vi "UpdateVariablesTC.vi"(8 "error in (no error)":errorcluster, 9 "SignificantDigits (8)":u32=8, 10 "Format (SI notation)":T1(ring)=enum."SI notation", 11 "VMUI in":refnum<class "VMUI.lvclass">) -> (0 "error out":errorcluster, 3 "VMUI out":refnum<class "VMUI.lvclass">)   [LabVIEW 2013, in "VMUI.lvclass"]
uses:
  VMUI.lvclass
  VariableManager/VariableManager.lvclass
  API/VariableManagerAPI.lvlib
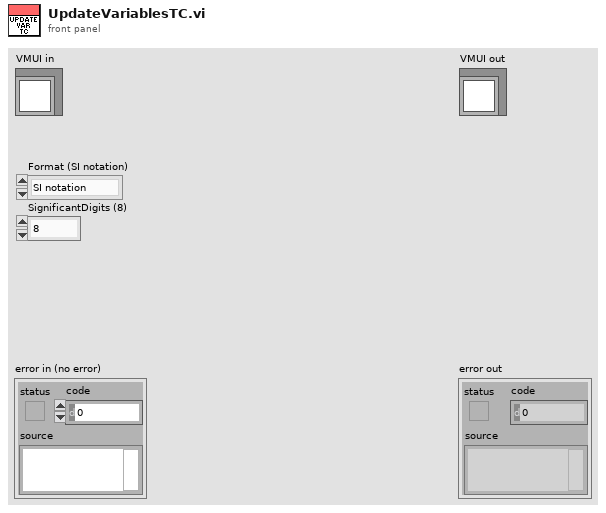
[diagram p1: front panel]
types:
  T1 = enum16{"Floating point", "Scientific SI", "Automatic SI", "SI notation"}
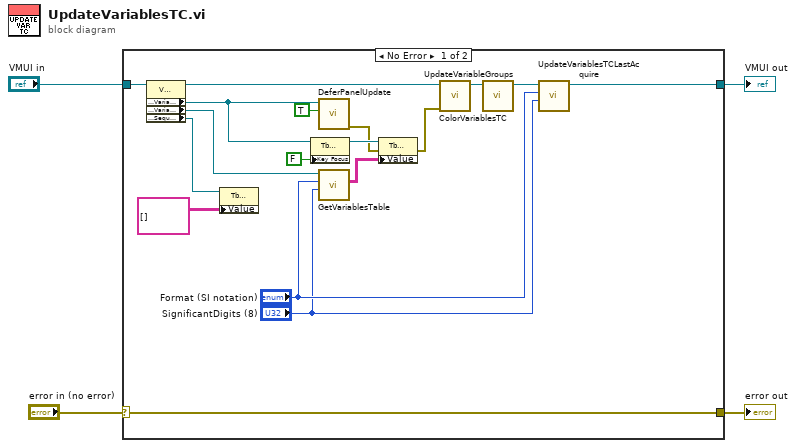
[diagram p0: block diagram]
diagram:
  n1 = case shown="No Error" "error in (no error)" {
    selector: "error in (no error)" -> [w21 w24]
    tunnel: [w21 w24] -> w3
    tunnel: [w7 w23] -> w1
    tunnel: "VMUI in" -> [w22 w23]
    frame No Error {
      n2 = property class="VMUI.lvclass"(reference=w22) -> (reference out=w17:refnum<class "VMUI.lvclass">, "Accessors:VariablesTCRef"=w12:refnum<vi>, "Accessors:VariableManagerRef"=w10:refnum<vi>, "Accessors:SequenceValuesTCRef"=w20:refnum<vi>)  [unwired: 1 in, 1 out]
      n3 = property class="Tbl (strict)"(reference=w20, "Value"=string[][] []) -> ()  [unwired: 1 in, 2 out]
      n4 = property class="Tbl (strict)"(reference=w12, "Key Focus"=FALSE) -> (reference out=w19:refnum<vi>)  [unwired: 1 in, 1 out]
      n5 = call "DeferPanelUpdate.vi"("Defer Panel Updates"=TRUE, "GObjectRefIn"=w12) -> ("error out"=w14:errorcluster)  [unwired: 9 in]
      n6 = call "GetVariablesTable.vi"("SignificantDigits (8)"="SignificantDigits (8)", "Format (SI notation)"="Format (SI notation)", "VariableManagerRef in"=w10) -> ("VariableTable"=w9:string[][])  [unwired: 6 in, 2 out]
      n7 = property class="Tbl (strict)"(reference=w19, error in=w14, "Value"=w9) -> (error out=w13:errorcluster)  [unwired: 1 out]
      n8 = call-dynamic "ColorVariablesTC.vi"("error in (no error)"=w13, "VMUI in"=w17) -> ("VMUI out"=w16:refnum<class "VMUI.lvclass">)  [unwired: 8 in, 1 out]
      n9 = call-dynamic "UpdateVariableGroups.vi"("VMUI in"=w16) -> ("VMUI out"=w8:refnum<class "VMUI.lvclass">)  [unwired: 9 in, 1 out]
      n10 = call-dynamic "UpdateVariablesTCLastAcquire.vi"("SignificantDigits (8)"="SignificantDigits (8)", "Format (SI notation)"="Format (SI notation)", "VMUI in"=w8) -> ("VMUI out"=w7:refnum<class "VMUI.lvclass">)  [unwired: 7 in, 1 out]
    }
    frame Error {
    }
  }
  "error out" <- w3
  "VMUI out" <- w1
